vi "deletePubKey.vi"(0 "HGF_GPG in":refnum<class "HGF_GPG.lvclass">, 1 "options file":path, 2 "keyringfile":path, 3 "Sec keyringfile":path, 5 "error in (no error)":errorcluster, 6 "key-id":string, 8 "Trust DB":path) -> (10 "dup Trust DB":path, 11 "success":bool, 12 "dup key-id":string, 14 "HGF_GPG out":refnum<class "HGF_GPG.lvclass">, 15 "dup options file":path, 16 "dup keyringfile":path, 17 "dup Sec keyringfile":path, 19 "error out":errorcluster)   [LabVIEW 2012, in "HGF_GPG.lvlib" / "HGF_GPG.lvclass"]
doc: "Delete the public key with Key-ID. If the secret key for this Id is installed you have to delete it first."
uses:
  HGF_GPG.lvclass
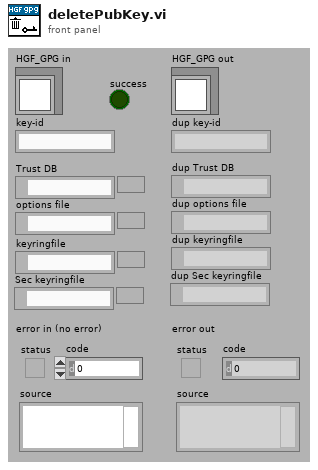
[diagram p1: front panel]
types:
  T1 = enum16{"list keys", "export", "import", "delete"}
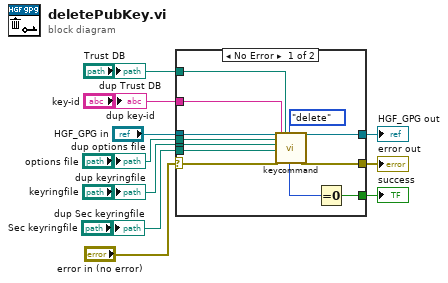
[diagram p0: block diagram]
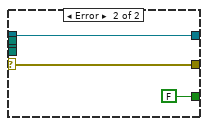
[diagram p2: hidden frame]
diagram:
  n1 = case shown="No Error" "error in (no error)" {
    selector: "error in (no error)" -> [w20 w25]
    tunnel: [w19 w25] -> w9
    tunnel: [w21 w24] -> w7
    tunnel: "HGF_GPG in" -> [w22 w24]
    tunnel: "key-id" -> [w14 _]
    tunnel: [w18 FALSE] -> w5
    tunnel: "keyringfile" -> [w17 _]
    tunnel: "options file" -> [w15 _]
    tunnel: "Sec keyringfile" -> [w13 _]
    tunnel: "Trust DB" -> [w12 _]
    frame No Error {
      n2 = call-dynamic "keycommand.vi"("HGF_GPG in"=w22, "options file"=w15, "keyringfile"=w17, "Sec keyringfile"=w13, "error in (no error)"=w20, "key-id"=w14, "Trust DB"=w12, "Enum"=T1."delete") -> ("return code"=w16:i32, "HGF_GPG out"=w21:refnum<class "HGF_GPG.lvclass">, "error out"=w19:errorcluster)  [unwired: 3 in, 14 out]
      n3 = Equal To 0?(x=w16) -> (x = 0?=w18:bool)
    }
    frame Error {
    }
  }
  "error out" <- w9
  "HGF_GPG out" <- w7
  "success" <- w5
  "dup options file" <- "options file"
  "dup keyringfile" <- "keyringfile"
  "dup key-id" <- "key-id"
  "dup Sec keyringfile" <- "Sec keyringfile"
  "dup Trust DB" <- "Trust DB"
